vi "Measure Resistance Only.vi"(6 "Published_ID":string="_Free", 7 "Settings":T2 {"Sense" items=["Local"=1008, "Remote"=1009]}, 8 "error in (no error)":errorcluster, 9 "current level":dbl format="%_6p", 10 "Pins":string[](array[string]), 11 "Semiconductor Module Context":T3) -> (0 "error out":errorcluster, 3 "Semiconductor Module Context Out":T3)   [LabVIEW 2013]
uses:
  <vilib>/NI_TestStand_SemiconductorModule/NI_TestStand_Semiconductor_Module.lvlibp/PinMap/General/SemiconductorModuleContext.ctl
  <instrlib>/niDCPower/nidcpower.llb/niDCPower Sense.ctl
  <instrlib>/niDCPower/nidcpower.llb/niDCPower Wait For Event - Event.ctl
  <vilib>/NI_TestStand_SemiconductorModule/NI_TestStand_Semiconductor_Module.lvlibp/PinMap/DC Power/PinToNIDCPowerSessions.vi
  <vilib>/NI_TestStand_SemiconductorModule/NI_TestStand_Semiconductor_Module.lvlibp/PinMap/General/Publish/PublishDataDoubleFunctionalTest.vi
  <vilib>/NI_TestStand_SemiconductorModule/NI_TestStand_Semiconductor_Module.lvlibp
panel:
  out "R Array":dbl[](array[numeric])
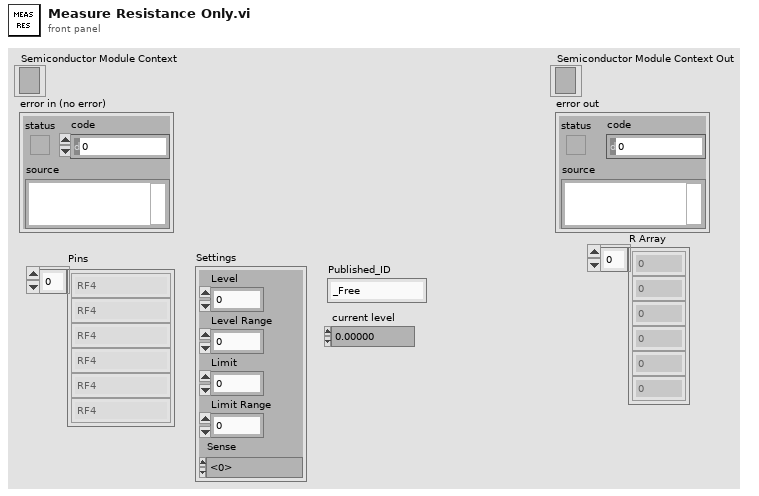
[diagram p1: front panel]
types:
  T1 = typedef "niDCPower Sense.ctl" = i32
  T2 = cluster{"Level":dbl, "Level Range":dbl, "Limit":dbl, "Limit Range":dbl, "Sense":T1}
  T3 = typedef "NI_TestStand_Semiconductor_Module.lvlibp/SemiconductorModuleContext.ctl" = refnum<k7>
  T4 = typedef "niDCPower Wait For Event - Event.ctl" = i32
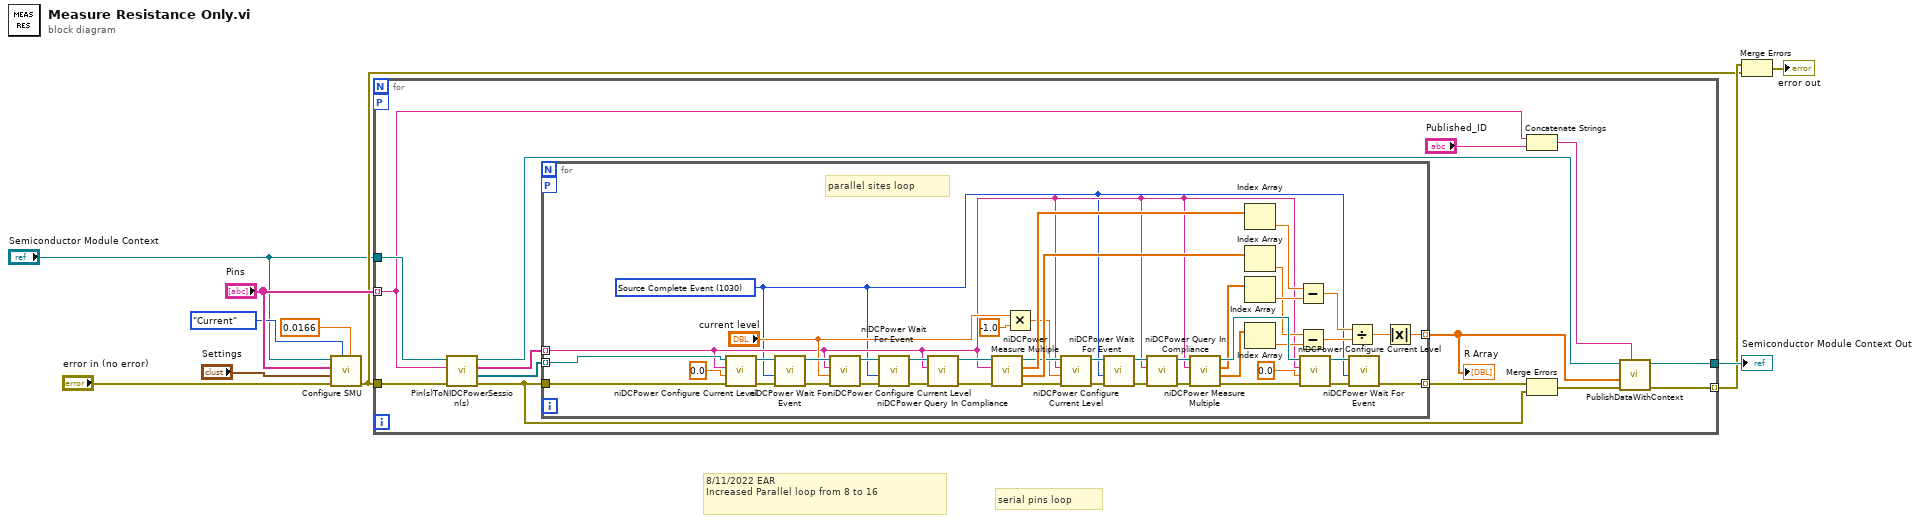
[diagram p0: block diagram]
diagram:
  # "8/11/2022 EAR\nIncreased Parallel loop from 8 to 16"
  # "serial pins loop"
  n1 = call "Configure SMU.vi"("aperture time"=0.0166, "Source Mode"=enum16{"Voltage", "Current"}."Current", "error in (no error)"="error in (no error)", "Settings"="Settings", "Pins"="Pins", "Semiconductor Module Context"="Semiconductor Module Context") -> ("error out"=w5:errorcluster)  [unwired: 5 in]
  n2 = for {
    tunnel: "Semiconductor Module Context" -> [w23]
    tunnel: [w17] -> w10
    tunnel: "Pins" -> [w14] mode=indexing
    tunnel: w5 -> [w24]
    tunnel: [w15] -> w8 mode=indexing
    workers-P: _ -> [_]
    n3 = call-poly <vilib>:"Pin(s)ToNIDCPowerSession(s).vi"("error in (no error)"=w24, "Pin"=w14, "Semiconductor Module Context"=w23) -> ("error out"=w19:errorcluster, "Instrument Sessions"=w21:refnum<k15>[], "Channel Lists"=w22:string[], "Semiconductor Module Context Out"=w18:T3)  [unwired: 4 in, 1 out]
    n4 = for {
      tunnel: w22 -> [w26] mode=indexing
      tunnel: w21 -> [w48] mode=indexing
      workers-P: _ -> [_]
      tunnel: w19 -> [w53]
      tunnel: [w66] -> w20 mode=indexing
      tunnel: [w55] -> w11 mode=indexing
      w25 = T4 1030 items=["Source Complete Event"=1030, "Measure Complete Event"=1031, "Sequence Iteration Complete Event"=1032, "Sequence Engine Done Event"=1033, "Pulse Complete Event"=1051, "Ready For Pulse Trigger Event"=1052] ("event")
      # "parallel sites loop"
      n5 = call <instrlib>:"niDCPower Configure Current Level.vi"("error in (no error)"=w53, "current level"=0.0, "channel name"=w26, "instrument handle"=w48) -> ("error out"=w52:errorcluster, "instrument handle out"=w50:refnum<k15>)  [unwired: 6 in]
      n6 = call <instrlib>:"niDCPower Wait For Event.vi"("error in (no error)"=w52, "event"=w25, "instrument handle"=w50) -> ("error out"=w51:errorcluster, "instrument handle out"=w49:refnum<k15>)  [unwired: 7 in]
      n7 = call <instrlib>:"niDCPower Configure Current Level.vi"("error in (no error)"=w51, "current level"="current level", "channel name"=w26, "instrument handle"=w49) -> ("error out"=w60:errorcluster, "instrument handle out"=w59:refnum<k15>)  [unwired: 6 in]
      n8 = call <instrlib>:"niDCPower Wait For Event.vi"("error in (no error)"=w60, "event"=w25, "instrument handle"=w59) -> ("error out"=w68:errorcluster, "instrument handle out"=w65:refnum<k15>)  [unwired: 7 in]
      n9 = call <instrlib>:"niDCPower Query In Compliance.vi"("error in (no error)"=w68, "channel name"=w26, "instrument handle"=w65) -> ("error out"=w61:errorcluster, "instrument handle out"=w62:refnum<k15>)  [unwired: 6 in, 1 out]
      n10 = call <instrlib>:"niDCPower Measure Multiple.vi"("error in (no error)"=w61, "channel name"=w26, "instrument handle"=w62) -> ("error out"=w39:errorcluster, "current measurements"=w56:dbl[], "voltage measurements"=w57:dbl[], "instrument handle out"=w37:refnum<k15>)  [unwired: 5 in]
      n11 = Multiply(x="current level", y=-1.0) -> (x*y=w27:dbl)
      n12 = call <instrlib>:"niDCPower Configure Current Level.vi"("error in (no error)"=w39, "current level"=w27, "channel name"=w26, "instrument handle"=w37) -> ("error out"=w42:errorcluster, "instrument handle out"=w41:refnum<k15>)  [unwired: 6 in]
      n13 = call <instrlib>:"niDCPower Wait For Event.vi"("error in (no error)"=w42, "event"=w25, "instrument handle"=w41) -> ("error out"=w40:errorcluster, "instrument handle out"=w45:refnum<k15>)  [unwired: 7 in]
      n14 = call <instrlib>:"niDCPower Query In Compliance.vi"("error in (no error)"=w40, "channel name"=w26, "instrument handle"=w45) -> ("error out"=w43:errorcluster, "instrument handle out"=w44:refnum<k15>)  [unwired: 6 in, 1 out]
      n15 = call <instrlib>:"niDCPower Measure Multiple.vi"("error in (no error)"=w43, "channel name"=w26, "instrument handle"=w44) -> ("error out"=w38:errorcluster, "current measurements"=w34:dbl[], "voltage measurements"=w35:dbl[], "instrument handle out"=w36:refnum<k15>)  [unwired: 5 in]
      n16 = Index Array(array=w57) -> (element=w33:dbl)  [unwired: 1 in]
      n17 = Index Array(array=w56) -> (element=w31:dbl)  [unwired: 1 in]
      n18 = Index Array(array=w35) -> (element=w32:dbl)  [unwired: 1 in]
      n19 = Index Array(array=w34) -> (element=w30:dbl)  [unwired: 1 in]
      n20 = Subtract(x=w33, y=w32) -> (x-y=w29:dbl)
      n21 = Subtract(x=w31, y=w30) -> (x-y=w28:dbl)
      n22 = call <instrlib>:"niDCPower Configure Current Level.vi"("error in (no error)"=w38, "current level"=0.0, "channel name"=w26, "instrument handle"=w36) -> ("error out"=w67:errorcluster, "instrument handle out"=w64:refnum<k15>)  [unwired: 6 in]
      n23 = Divide(x=w29, y=w28) -> (x/y=w58:dbl)
      n24 = call <instrlib>:"niDCPower Wait For Event.vi"("error in (no error)"=w67, "event"=w25, "instrument handle"=w64) -> ("error out"=w66:errorcluster)  [unwired: 7 in, 1 out]
      n25 = Absolute Value(x=w58) -> (abs(x)=w55:dbl)
    }
    "R Array" <- w11
    n26 = Concatenate Strings(w14, "Published_ID") -> (w12:string)
    n27 = Merge Errors(w20, w19) -> (w16:errorcluster)
    n28 = call-poly <vilib>:"PublishDataWithContext.vi"("Published Data Id"=w12, "error in (no error)"=w16, "Data In"=w11, "Semiconductor Module Context"=w18) -> ("error out"=w15:errorcluster, "Semiconductor Module Context Out"=w17:T3)  [unwired: 6 in]
  }
  "Semiconductor Module Context Out" <- w10
  n29 = Merge Errors(w8, w5) -> (→"error out":errorcluster)
